vi "sv_Get Index for Unit label.vi"(11 "measurement selection":bool[](array[boolean])) -> (3 "index":i32)   [LabVIEW 2017]
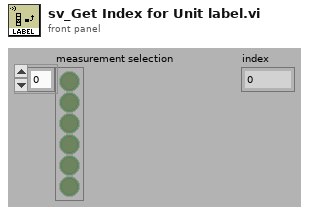
[diagram p1: front panel]
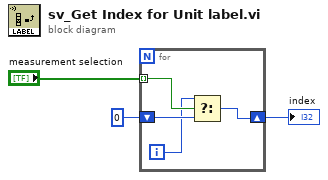
[diagram p0: block diagram]
diagram:
  n1 = for {
    tunnel: "measurement selection" -> [w7] mode=indexing
    shift-right: [w4] -> w1
    shift-left: 0 ("index") -> [w6]
    i -> [w5]
    n2 = Select(t=w5, s=w7, f=w6) -> (s? t:f=w4:i32)
  }
  "index" <- w1
